vi "Print Image from Microsoft Paint.vi"(8 "error out":errorcluster, 11 "Path to PNG File":path) -> (0 "error out":errorcluster)   [LabVIEW 2011]
panel:
  # "This VI programmatically calls Microsoft paint to print a PNG file to your default printer."
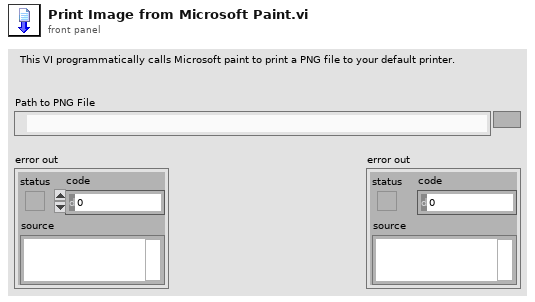
[diagram p1: front panel]
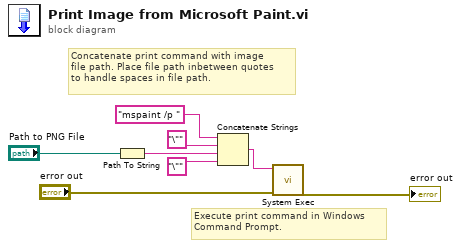
[diagram p0: block diagram]
diagram:
  # "Concatenate print command with image \nfile path. Place file path inbetween quotes \nto handle spaces in file path."
  # "Execute print command in Windows\nCommand Prompt."
  n1 = Path To String(path="Path to PNG File") -> (string=w3:string)
  n2 = Concatenate Strings("mspaint /p " ("command line"), "\"" ("string"), w3, "\"" ("string")) -> (w6:string)
  n3 = call <vilib>:"System Exec.vi"("error in (no error)"="error out", "command line"=w6) -> ("error out"=→"error out":errorcluster)  [unwired: 6 in, 3 out]
